vi "SVM_Train_FromFile.vi"() -> (0 "error out":errorcluster)   [LabVIEW 2014]
uses:
  Controls/Kernel.ctl
  Libsvm Wrapper/Controls/svm_kernel_type.ctl
  Controls/Options Training.ctl
  Controls/Parameters NU_SVC.ctl
  Libsvm Wrapper/Controls/svm_model.ctl
  Libsvm Wrapper/Controls/svm_parameter.ctl
  Libsvm Wrapper/Controls/svm_type.ctl
  Libsvm Wrapper/Controls/svm_node.ctl
  Logger/Controls/GFV Action.ctl
  SubVIs/SVM Train NU_SVC.vi
  <userlib>/_OpenG.lib/error/error.llb/Filter Error Codes (Array)__ogtk.vi
  Libsvm Wrapper/svm_train.vi
  Libsvm Wrapper/svm_predict.vi
panel:
  out "Model":T1
  out "N Predicted":i16
  out "N Nodes":i32
  in  "nu":T6=0.2 caption="nu (0,5)"
  in  "Options":T7={"cache_size"=500.0, "eps"=0.001, "shrinking"=TRUE, "probability"=FALSE}
  in  "Kernel":T8
  out "Logging output":string
  # "Test set"
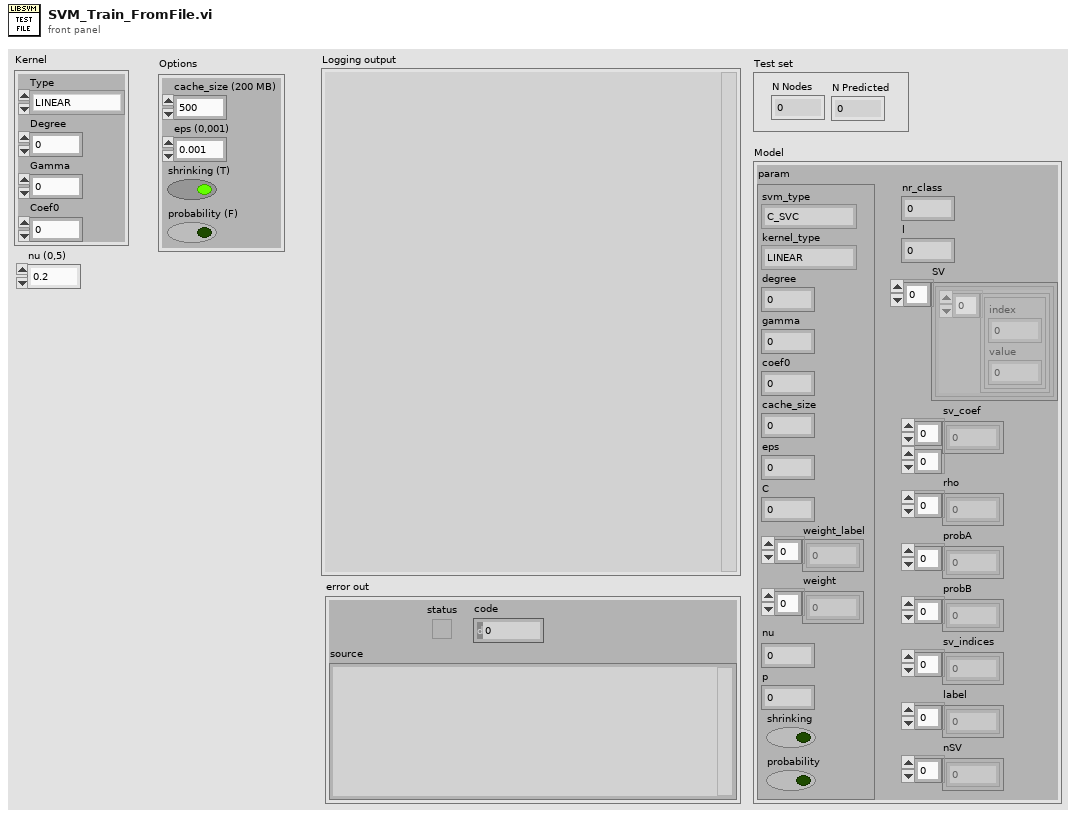
[diagram p1: front panel]
types:
  T1 = typedef "svm_model.ctl" = cluster{"param":T2, "nr_class":i32, "l":i32, "SV":cluster{"Array":T5[]}[], "sv_coef":dbl[][], "rho":dbl[], "probA":dbl[], "probB":dbl[], "sv_indices":i32[], "label":i32[], "nSV":i32[]}
  T2 = typedef "svm_parameter.ctl" = cluster{"svm_type":T3, "kernel_type":T4, "degree":i32, "gamma":dbl, "coef0":dbl, "cache_size":dbl, "eps":dbl, "C":dbl, "weight_label":i32[], "weight":dbl[], "nu":dbl, "p":dbl, "shrinking":bool, "probability":bool}
  T3 = typedef "svm_type.ctl" = enum32{"C_SVC", "NU_SVC", "ONE_CLASS", "EPSILON_SVR", "NU_SVR"}
  T4 = typedef "svm_kernel_type.ctl" = enum32{"LINEAR", "POLY", "RBF", "SIGMOID", "PRECOMPUTED"}
  T5 = typedef "svm_node.ctl" = cluster{"index":i32, "value":dbl}
  T6 = typedef "Parameters NU_SVC.ctl" = dbl
  T7 = typedef "Options Training.ctl" = cluster{"cache_size":dbl, "eps":dbl, "shrinking":bool, "probability":bool}
  T8 = typedef "Kernel.ctl" = cluster{"Type":T4, "Degree":i32, "Gamma":dbl, "Coef0":dbl}
  T9 = typedef "GFV Action.ctl" = enum16{"Get", "Set", "Delete"}
  T10 = typedef "Logging_MessageQueue.ctl" = cluster{"Time":timestamp, "message":string}
  T11 = typedef "svm_problem.ctl" = cluster{"y":dbl[], "x":cluster{T5[]}[]}
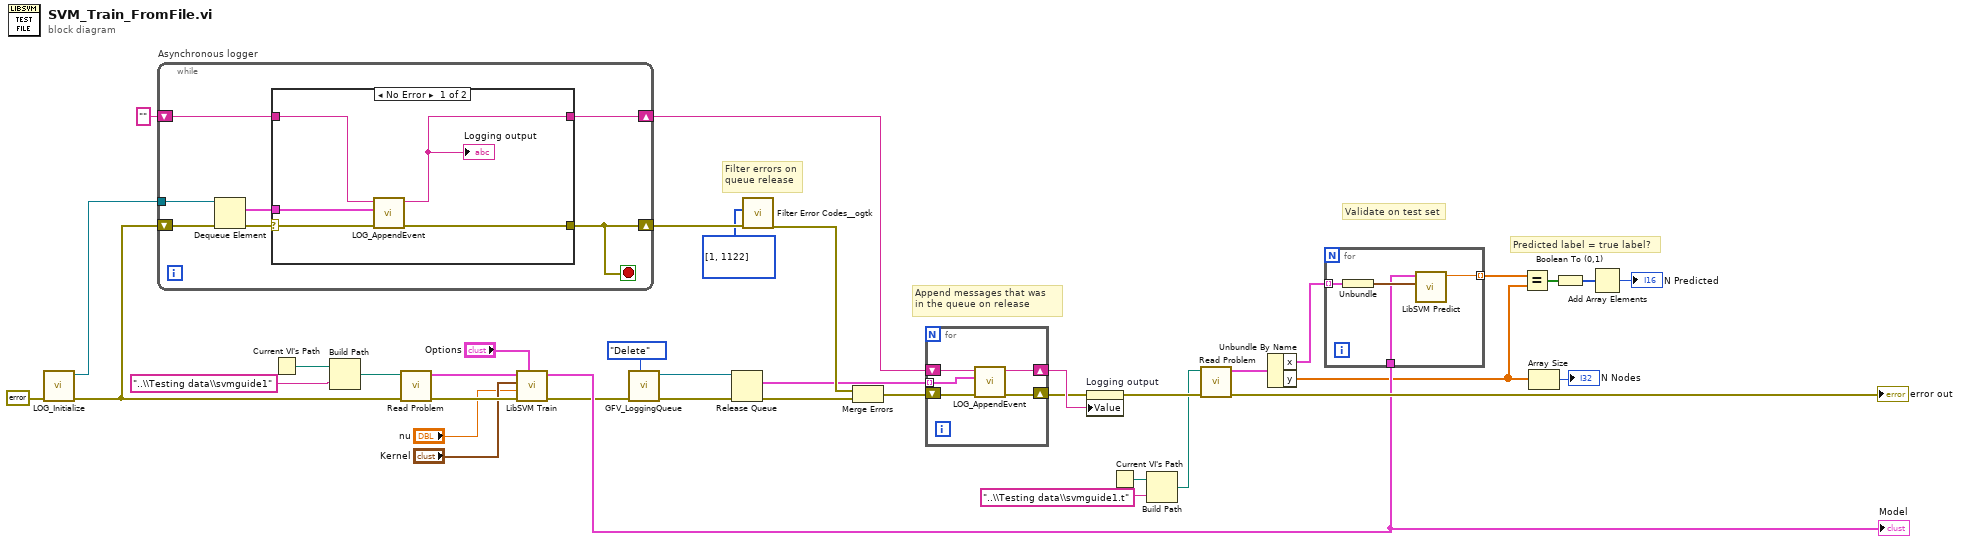
[diagram p0: block diagram]
diagram:
  # "Predicted label = true label?"
  # "Validate on test set"
  # "Append messages that was \nin the queue on release"
  # "Filter errors on\nqueue release"
  n1 = call "LOG_Initialize.vi"("error in (no error)"=errorcluster {"status"=FALSE, "code"=0, "source"=""} ("error IO")) -> ("error out"=w33:errorcluster, "Message queue out"=w34:refnum<queue>)  [unwired: 9 in]
  n2 = while "Asynchronous logger" {
    tunnel: w34 -> [w46]
    shift-right: [w43] -> w26
    shift-left: "" -> [w42]
    shift-right: [w40] -> w31
    shift-left: w33 -> [w44]
    stop <- w40 stop-if-true
    n3 = Dequeue Element(queue=w46, error in (no error)=w44) -> (element=w45:T10, error out=w41:errorcluster)  [unwired: 1 in, 2 out]
    n4 = case shown="No Error" w41 {
      selector: w41 -> [w48 w53]
      tunnel: w45 -> [w51 _]
      tunnel: [w50 w52] -> w43
      tunnel: w42 -> [w49 w52]
      tunnel: [w47 w53] -> w40
      frame No Error {
        n5 = call "LOG_AppendEvent.vi"("error in (no error)"=w48, "Log Event"=w51, "String in"=w49) -> ("error out"=w47:errorcluster, "String out"=w50:string)  [unwired: 7 in]
        "Logging output" <- w50
      }
      frame Error {
      }
    }
  }
  n6 = Current VI's Path() -> (path=w14:path)
  n7 = Build Path(base path=w14, name or relative path="..\\Testing data\\svmguide1") -> (appended path=w36:path)
  n8 = call "Read Problem.vi"("error in (no error)"=w33, "file path (use dialog)"=w36) -> ("error out"=w18:errorcluster, "svm_problem"=w20:T11)  [unwired: 8 in]
  n9 = call-poly "LibSVM Train.vi"("Options"="Options", "error in (no error)"=w18, "nu"="nu", "Kernel"="Kernel", "Problem"=w20) -> ("error out"=w19:errorcluster, "Model"=w38:T1)  [unwired: 5 in]
  "Model" <- w38
  n10 = call "GFV_LoggingQueue.vi"("GFV Action"=GFV_Action."Delete", "error in (no error)"=w19) -> ("error out"=w23:errorcluster, "Message queue out"=w22:refnum<queue>)  [unwired: 8 in]
  n11 = Release Queue(queue=w22, error in (no error)=w23) -> (remaining elements=w28:T10[], error out=w32:errorcluster)  [unwired: 1 in, 1 out]
  n12 = call-poly <userlib>:"Filter Error Codes__ogtk.vi"("Error In"=w31, "Error Codes to Filter"=i32[] [1, 1122]) -> ("Error Out"=w30:errorcluster)  [unwired: 7 in, 2 out]
  n13 = Merge Errors(w30, w32) -> (w27:errorcluster)
  n14 = for {
    tunnel: w28 -> [w57] mode=indexing
    shift-right: [w55] -> w24
    shift-left: w27 -> [w58]
    shift-right: [w54] -> w25
    shift-left: w26 -> [w56]
    n15 = call "LOG_AppendEvent.vi"("error in (no error)"=w58, "Log Event"=w57, "String in"=w56) -> ("error out"=w55:errorcluster, "String out"=w54:string)  [unwired: 7 in]
  }
  n16 = property on="Logging output" class="Str"(error in=w24, "Value"=w25) -> (error out=w7:errorcluster)  [unwired: 1 in, 1 out]
  n17 = Current VI's Path() -> (path=w5:path)
  n18 = Build Path(base path=w5, name or relative path="..\\Testing data\\svmguide1.t") -> (appended path=w4:path)
  n19 = call "Read Problem.vi"("error in (no error)"=w7, "file path (use dialog)"=w4) -> ("error out"=→"error out":errorcluster, "svm_problem"=w12:T11)  [unwired: 8 in]
  n20 = Unbundle By Name(w12) -> ("x"=w11:cluster{T5[]}[], "y"=w9:dbl[])
  n21 = for {
    tunnel: w11 -> [w62] mode=indexing
    tunnel: [w60] -> w10 mode=indexing
    tunnel: w38 -> [w59]
    n22 = Unbundle(w62) -> (w61:T5[])
    n23 = call-poly "LibSVM Predict.vi"("X"=w61, "Model"=w59) -> ("Predicted label"=w60:dbl)  [unwired: 8 in, 1 out]
  }
  n24 = Equal?(x=w10, y=w9) -> (x = y?=w3:bool[])
  n25 = Array Size(array=w9) -> (size(s)=→"N Nodes":i32)
  n26 = Boolean To (0,1)(Boolean=w3) -> (0, 1=w2:i16[])
  n27 = Add Array Elements(numeric array=w2) -> (sum=→"N Predicted":i16)
